vi "Remote APIs for base station configuration GET.vi"() -> ()   [LabVIEW 2021]
uses:
  Controls/TCP_FGV.ctl
  Controls/Cellular_Technology.ctl
panel:
  in  "error in (no error)":errorcluster
  out "error out":errorcluster
  in  "Option":string
  in  "Base Station":T1
  in  "Cellular Technology":T1
  in  "UE_ID":i32
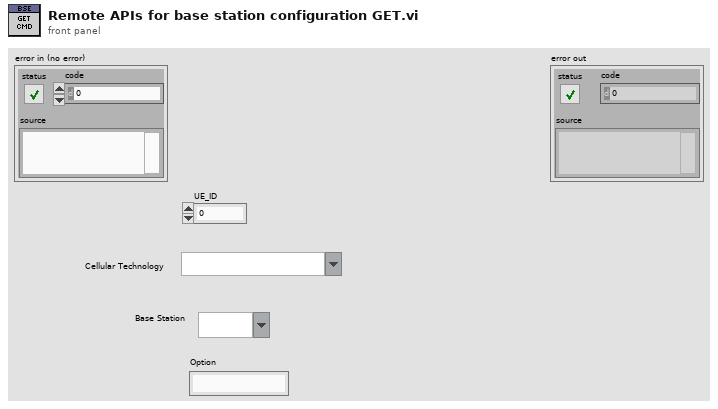
[diagram p1: front panel]
types:
  T1 = typedef "Cellular_Technology.ctl" = string
  T2 = typedef "TCP_FGV.ctl" = enum16{"Open", "Read", "Write", "Close"}
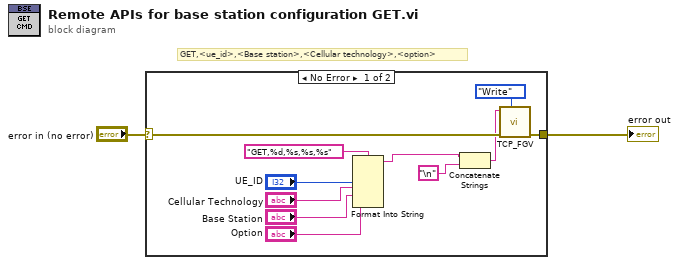
[diagram p0: block diagram]
diagram:
  # "GET,<ue_id>,<Base station>,<Cellular technology>,<option>"
  n1 = case shown="No Error" "error in (no error)" {
    selector: "error in (no error)" -> [w7 w14]
    tunnel: [w8 w14] -> w2
    frame No Error {
      n2 = Format Into String(format string="GET,%d,%s,%s,%s", "UE_ID", "Cellular Technology", "Base Station", "Option") -> (resulting string=w4:string)  [unwired: 2 in, 1 out]
      n3 = Concatenate Strings(w4, "\n") -> (w3:string)
      n4 = call "TCP_FGV.vi"("Command"=w3, "error in (no error)"=w7, "Operation"=TCP_FGV."Write") -> ("error out"=w8:errorcluster)  [unwired: 6 in, 1 out]
    }
    frame Error {
    }
  }
  "error out" <- w2
